vi "Total Mean Angle (SubVI).vi"(9 "Angle Valid":bool, 10 "Angle":fxp<+/-,16,3> format="%.14g", 11 "Done In":bool) -> (0 "Mean Angle":fxp<+/-,32,16> format="%.14g", 3 "Done Out":bool)   [LabVIEW 2015]
uses:
  <vilib>/rvi/FXPMathLib/FxpDiv/subVIs/nifxpmath_Div_SimConfig.ctl
  <vilib>/rvi/FXPMathLib/FxpDiv/simVIs/DllFxpDivTemp_sub.vi
  <vilib>/rvi/FXPMathLib/FxpDiv/XNode/nifxpmath_Div.xnode
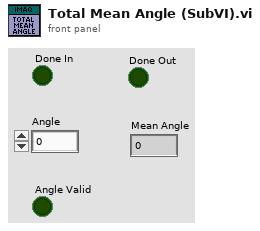
[diagram p1: front panel]
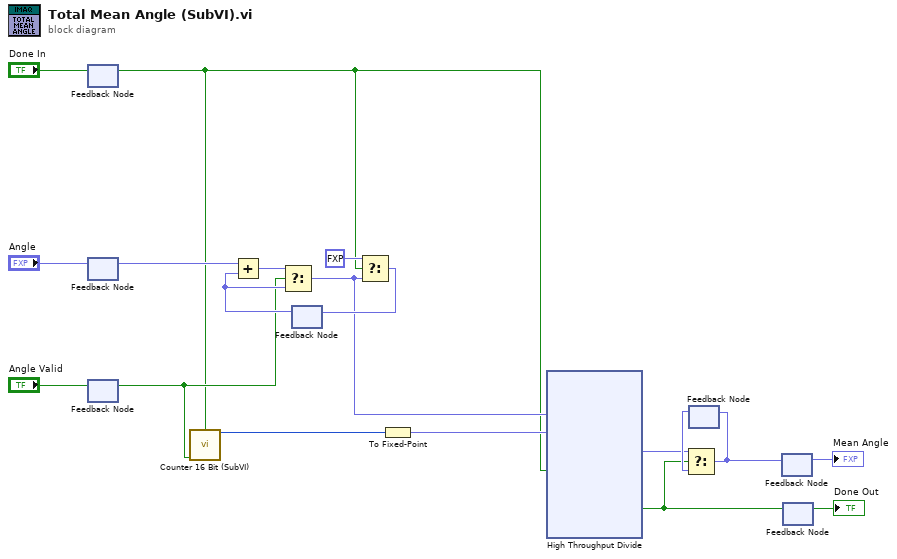
[diagram p0: block diagram]
diagram:
  n1 = feedback-in #1("Done In") -> ()
  n2 = feedback #1() -> (w6:bool)  [unwired: 1 in]
  n3 = feedback-in #2("Angle") -> ()
  n4 = feedback #2() -> (w15:fxp<+/-,16,3>)  [unwired: 1 in]
  n5 = feedback-in #3("Angle Valid") -> ()
  n6 = feedback #3() -> (w10:bool)  [unwired: 1 in]
  n7 = call "Counter 16 Bit (SubVI).vi"("RESET"=w6, "Enable"=w10) -> ("Count"=w8:u16)  [unwired: 11 in, 2 out]
  n8 = feedback #4() -> (w11:fxp<+/-,32,16>)  [unwired: 1 in]
  n9 = Add(x=w15, y=w11) -> (x+y=w12:fxp<+/-,32,16>)
  n10 = Select(t=w12, s=w10, f=w11) -> (s? t:f=w9:fxp<+/-,32,16>)
  n11 = Select(t=fxp<+/-,32,16> 0.0, s=w6, f=w9) -> (s? t:f=w14:fxp<+/-,32,16>)
  n12 = feedback-in #4(w14) -> ()
  n13 = To Fixed-Point(number=w8) -> (fixed-point=w7:fxp<+/-,16,16>)  [unwired: 1 in]
  n14 = xnode "High Throughput Divide"("x"=w9, "y"=w7, "input valid"=w6) -> ("x/y"=w3:fxp<+/-,32,16>, "output valid"=w1:bool)  [unwired: 1 in, 1 out]
  n15 = feedback #5() -> (w4:fxp<+/-,32,16>)  [unwired: 1 in]
  n16 = Select(t=w3, s=w1, f=w4) -> (s? t:f=w2:fxp<+/-,32,16>)
  n17 = feedback-in #5(w2) -> ()
  n18 = feedback #6() -> (→"Mean Angle":fxp<+/-,32,16>)  [unwired: 1 in]
  n19 = feedback-in #6(w2) -> ()
  n20 = feedback #7() -> (→"Done Out":bool)  [unwired: 1 in]
  n21 = feedback-in #7(w1) -> ()
